vi "Global_SIM_switch.vi"() -> ()   [LabVIEW 2016]
panel:
  in  "enable_IKMGS_file":bool=TRUE
  in  "enable_YSI_file":bool=TRUE
  in  "enable_kpro_file":bool=TRUE
  in  "enable_slug_file":bool=TRUE
  in  "use_kpro_file_only":bool=TRUE
  in  "Simulate AD6B":bool
  # "ON"
  # "ON"
  # "OFF"
  # "OFF"
  # "ON"
  # "ON"
  # "ON"
  # "ON"
  # "OFF"
  # "OFF"
  # "OFF"
  # "OFF"
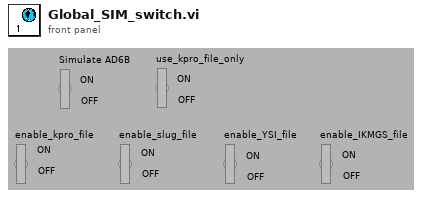
[diagram p1: front panel]
diagram:
